vi "Build Report String.vi"(8 "error in (no error)":errorcluster, 10 "Result":T1, 11 "String Assertion in":refnum<class "String Assertion.lvclass">) -> (0 "error out":errorcluster, 2 "Report String":string, 3 "String Assertion out":refnum<class "String Assertion.lvclass">)   [LabVIEW 2020, in "MacroAssert.lvlib" / "String Assertion.lvclass"]
doc: "Builds a string using <B>Step</B> and <B>Result</B> to be included in a report."
uses:
  String Assertion.lvclass
  String Assertion.lvclass/String Assertion.ctl
  MacroAssert.lvlib
  CTLs/Result.ctl
  CTLs/Outcome.ctl
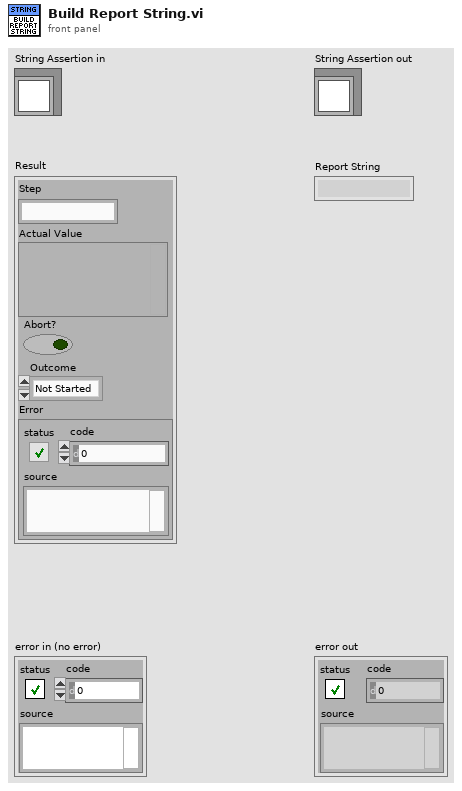
[diagram p1: front panel]
types:
  T1 = typedef "MacroAssert.lvlib/Result.ctl" = cluster{"Step":string, "Actual Value":variant, "Abort?":bool, "Outcome":T2, "Error":errorcluster}
  T2 = typedef "MacroAssert.lvlib/Outcome.ctl" = enum16{"Not Started", "Skipped", "Pass", "Fail", "Complete", "Error", "Auto Abort", "User Abort"}
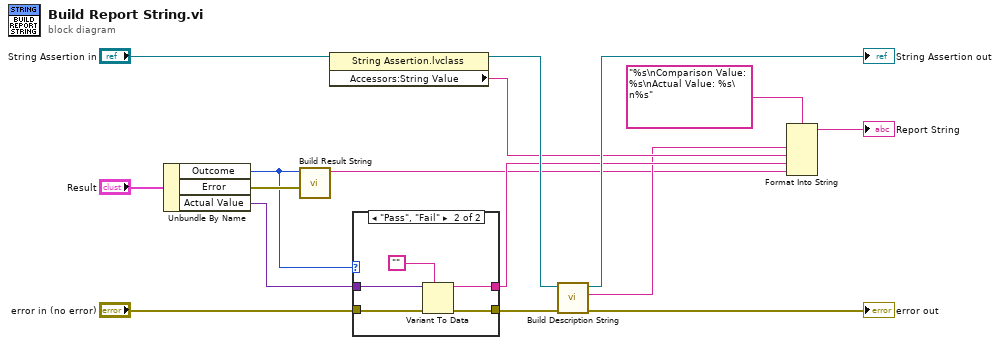
[diagram p0: block diagram]
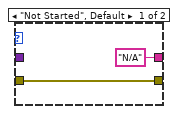
[diagram p2: hidden frame]
diagram:
  n1 = Unbundle By Name("Result") -> ("Outcome"=w2:T2, "Error"=w13:errorcluster, "Actual Value"=w9:variant)
  n2 = call "Build Result String.vi"("Error"=w13, "Outcome"=w2) -> ("Result String"=w1:string)  [unwired: 9 in]
  n3 = property class="String Assertion.lvclass"(reference="String Assertion in") -> (reference out=w6:refnum<class "String Assertion.lvclass">, "Accessors:String Value"=w4:string)  [unwired: 1 in, 1 out]
  n4 = case shown="\"Pass\", \"Fail\"" w2 {
    tunnel: w9 -> [_ w21]
    tunnel: "error in (no error)" -> [w18 w23]
    tunnel: [w18 w22] -> w14
    tunnel: ["N/A" w19] -> w5
    frame "Not Started", Default {
    }
    frame "Pass", "Fail" {
      n5 = Variant To Data(error in=w23, type="", Variant=w21) -> (data=w19:string, error out=w22:errorcluster)
    }
  }
  n6 = call-dynamic "Build Description String.vi"("error in (no error)"=w14, "String Assertion in"=w6) -> ("error out"=→"error out":errorcluster, "Description"=w3:string, "String Assertion out"=→"String Assertion out":refnum<class "String Assertion.lvclass">)  [unwired: 7 in]
  n7 = Format Into String(format string="%s\nComparison Value: %s\nActual Value: %s\n%s", w3, w4, w5, w1) -> (resulting string=→"Report String":string)  [unwired: 2 in, 1 out]
